vi "GetGrayScale.vi"(8 "error in (no error)":errorcluster, 11 "ColorGrayScale in":refnum<class "ColorGrayScale.lvclass">) -> (0 "error out":errorcluster, 2 "Color":u32(colorbox), 3 "ColorGrayScale out":refnum<class "ColorGrayScale.lvclass">)   [LabVIEW 2021, in "Picture2D.lvlib" / "ColorGrayScale.lvclass"]
uses:
  ColorGrayScale.lvclass
  ColorRGBA/ColorRGBA.lvclass
  ColorGrayScale.lvclass/ColorGrayScale.ctl
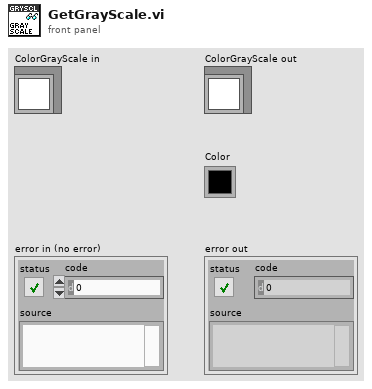
[diagram p1: front panel]
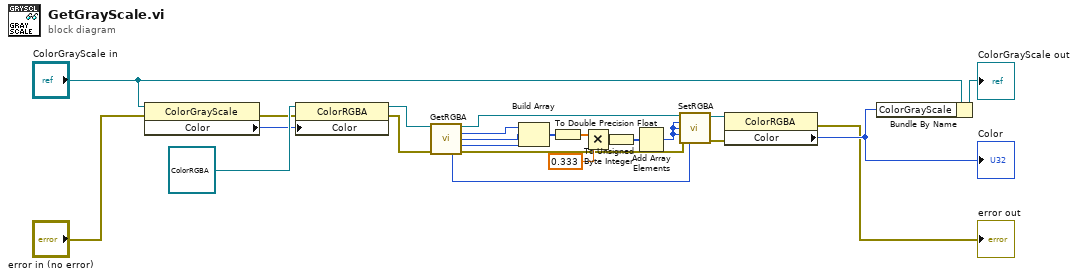
[diagram p0: block diagram]
diagram:
  n1 = property class="ColorGrayScale"(reference="ColorGrayScale in", error in="error in (no error)") -> (error out=w2:errorcluster, "Color"=w15:u32)  [unwired: 1 out]
  n2 = property class="ColorRGBA"(reference=refnum<class "ColorRGBA.lvclass"> refnum ("Picture2D.lvlib:ColorRGBA"), error in=w2, "Color"=w15) -> (reference out=w14:refnum<class "ColorRGBA.lvclass">, error out=w13:errorcluster)
  n3 = call-dynamic "GetRGBA.vi"("ColorRGBA in"=w14, "error in (no error)"=w13) -> ("ColorRGBA out"=w9:refnum<class "ColorRGBA.lvclass">, "R"=w12:u8, "G"=w11:u8, "B"=w10:u8, "A"=w7:u8, "error out"=w6:errorcluster)  [unwired: 8 in]
  n4 = Build Array(w12, w11, w10) -> (w22:u8[])
  n5 = To Double Precision Float(number=w22) -> (double precision float=w19:dbl[])
  n6 = Multiply(x=w19, y=0.333) -> (x*y=w20:dbl[])
  n7 = To Unsigned Byte Integer(number=w20) -> (unsigned 8bit integer=w17:u8[])
  n8 = Add Array Elements(numeric array=w17) -> (sum=w8:u8)
  n9 = call-dynamic "SetRGBA.vi"("ColorRGBA in"=w9, "R"=w8, "G"=w8, "B"=w8, "error in (no error)"=w6, "A"=w7) -> ("ColorRGBA out"=w5:refnum<class "ColorRGBA.lvclass">, "error out"=w3:errorcluster)  [unwired: 8 in]
  n10 = property class="ColorRGBA"(reference=w5, error in=w3) -> (error out=→"error out":errorcluster, "Color"=w4:u32)  [unwired: 1 out]
  "Color" <- w4
  n11 = Bundle By Name(cluster="ColorGrayScale in", "ColorGrayScale"=w4) -> (→"ColorGrayScale out":refnum<class "ColorGrayScale.lvclass">)
